vi "Custom Automation Tool.vi"(8 "error in (no error)":errorcluster) -> (0 "error out":errorcluster)   [LabVIEW 2023]
doc: "Presents an interface to either update a specification limit, or add a new one."
uses:
  CTLs/Step.ctl
  CTLs/Step Type.ctl
  <vilib>/Utility/config.llb/Config Data RefNum.ctl
  <vilib>/Utility/miscctls.llb/LVRowAndColumnUnsignedTypeDef.ctl
  CTLs/FGV Actions.ctl
  bd503c13-d10c-440e-ab5e-4e60baef5deb.vi
  cc7d3372-ed48-481f-8659-91fce09351ce.vi
  <vilib>/Utility/config.llb/Write Key (String).vi
  <vilib>/Utility/config.llb/Read Key (String).vi
  <userlib>/_MGI/Application Control/MGI Gray if/MGI Gray if False.vi
  <vilib>/Utility/inputDevices.llb/keyboardAcquire.vi
  <vilib>/Utility/inputDevices.llb/closeKeyboard.vi
  <vilib>/Utility/config.llb/NI_LVConfig.lvlib
  SubVIs/FaKI State Machine/FaKI State Machine.lvlib
panel:
  in  "Settings":bool
  in  "Export":bool
  in  "Import":bool
  out "Application Hotkey":string
  in  "Delete":bool
  in  "Start/Stop":bool
  in  "N":i32 caption="Times to Repeat\n(-1 = indefinitely)" min=-1
  in  "Activation Type":enum32{"Hotkey", "Automatic"}(radio)
  out "Menu":bool
  out "Row":i32
  in  "Add Step 2":bool
  in  "Dbl Click":T1
  out "Table":string[][](table)
  in  "Clear Profile":bool
  in  "Delete Step":bool
  in  "Insert Step":bool
  in  "Add Step":bool
  in  "Modify Step":bool
  in  "Close":bool
  in  "Save":bool
  in  "Restore":bool
  in  "Help":bool
  in  "Macro Name":string(combo)
  # "Table has double-click functionality"
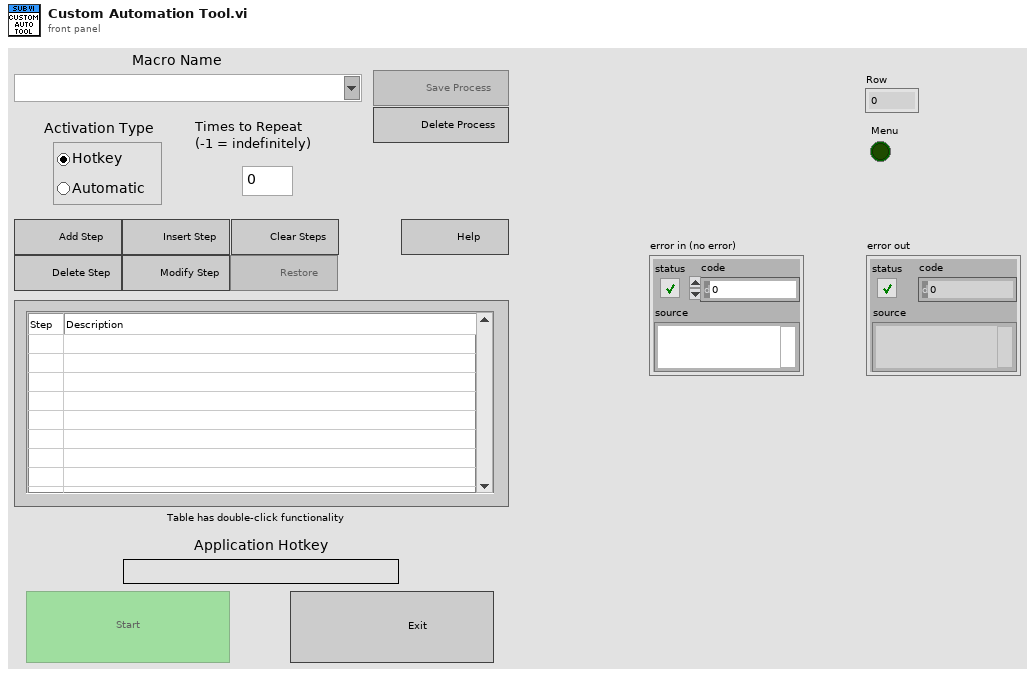
[diagram p1: front panel]
types:
  T1 = cluster{"Insert Before":bool, "Insert After":bool, "Modify":bool, "Delete":bool}
  T2 = typedef "LVPoint32TypeDef.ctl" = cluster{"Horizontal":i32, "Vertical":i32}
  T3 = typedef "LVRowAndColumnTypeDef.ctl" = cluster{"Row":i32, "Column":i32}
  T4 = enum32{"Invalid", "Standard", "Closed", "Hidden", "Minimized", "Maximized"}
  T5 = enum32{"invalid app kind", "Development System", "Run Time System", "Student Edition", "Embedded LabVIEW", "Evaluation", "Custom"}
  T6 = enum8{"Enabled", "Disabled", "Disabled and Grayed Out"}
  T7 = typedef "Step.ctl" = cluster{"Type":T8, "Coords":cluster{"x":i32, "y":i32}, "Delay":i32, "Key":u8, "Repeat":i32, "RClick?":bool}
  T8 = typedef "Step Type.ctl" = enum16{"Mouse Move", "Mouse Click", "Key Press", "Wait", "Mouse Down", "Mouse Up", "Key Down", "Key Up"}
  T9 = typedef "LVRowAndColumnUnsignedTypeDef.ctl" = cluster{"Row":u32, "Column":u32}
  T10 = cluster{"Steps":T7[], "Activation Type":enum32{"Hotkey", "Automatic"}, "N":i32}
  T11 = typedef "FGV Actions.ctl" = enum16{"Read", "Write"}
  T12 = typedef "NI_LVConfig.lvlib/Config Data RefNum.ctl" = refnum<k1>
  T13 = cluster{"Core":cluster{"Current VI Reference":refnum<vi>, "Close Panel on Exit?":bool}, "Steps":T7[], "Refs":refnum<vi>[], "Config":T12, "Step":i32, "n":i32, "Hotkey":enum16{"0", "1", "2", "3", "4", "5", "6", "7", "8", "9", "A", "B", "C", "D", "E", "F", "G", "H", "I", "J", "K", "L", "M", "N", "O", "P", "Q", "R", "S", "T", "U", "V", "W", "X", "Y", "Z", "F1", "F2", "F3", "F4", "F5", "F6", "F7", "F8", "F9", "F10", "F11", "F12", "F13", "F14", "F15", "ADD", "BACK", "BACKSLASH", "CAPITAL", "COMMA", "DECIMAL", "DELETE", "DIVIDE", "DOWN", "END", "EQUALS", "ESCAPE", "GRAVE (`)", "HOME", "INSERT", "LBRACKET", "LCONTROL", "LEFT", "L ALT", "LSHIFT", "LWIN", "MINUS", "MULTIPLY", "NEXT", "NUMLOCK", "NUMPAD_0", "NUMPAD_1", "NUMPAD_2", "NUMPAD_3", "NUMPAD_4", "NUMPAD_5", "NUMPAD_6", "NUMPAD_7", "NUMPAD_8", "NUMPAD_9", "PAUSE", "PERIOD", "PRIOR (PG UP)", "RBRACKET", "RCONTROL", "RETURN", "RIGHT", "R ALT", "RSHIFT", "RWIN", "SCROLL", "SEMICOLON", "SLASH", "SPACE", "SUBTRACT", "TAB", "UP", "ENTER (num pad)", "' (quote)"}[], "FP CTLs":cluster{"Name":string, "Type":enum32{"Hotkey", "Automatic"}, "N":i32}, "Keyboard":refnum<k1>}
  T14 = cluster{"Name":string, "Type":enum32{"Hotkey", "Automatic"}, "N":i32}
  T15 = enum16{"0", "1", "2", "3", "4", "5", "6", "7", "8", "9", "A", "B", "C", "D", "E", "F", "G", "H", "I", "J", "K", "L", "M", "N", "O", "P", "Q", "R", "S", "T", "U", "V", "W", "X", "Y", "Z", "F1", "F2", "F3", "F4", "F5", "F6", "F7", "F8", "F9", "F10", "F11", "F12", "F13", "F14", "F15", "ADD", "BACK", "BACKSLASH", "CAPITAL", "COMMA", "DECIMAL", "DELETE", "DIVIDE", "DOWN", "END", "EQUALS", "ESCAPE", "GRAVE (`)", "HOME", "INSERT", "LBRACKET", "LCONTROL", "LEFT", "L ALT", "LSHIFT", "LWIN", "MINUS", "MULTIPLY", "NEXT", "NUMLOCK", "NUMPAD_0", "NUMPAD_1", "NUMPAD_2", "NUMPAD_3", "NUMPAD_4", "NUMPAD_5", "NUMPAD_6", "NUMPAD_7", "NUMPAD_8", "NUMPAD_9", "PAUSE", "PERIOD", "PRIOR (PG UP)", "RBRACKET", "RCONTROL", "RETURN", "RIGHT", "R ALT", "RSHIFT", "RWIN", "SCROLL", "SEMICOLON", "SLASH", "SPACE", "SUBTRACT", "TAB", "UP", "ENTER (num pad)", "' (quote)"}[]
  T16 = cluster{"Current VI Reference":refnum<vi>, "Close Panel on Exit?":bool}
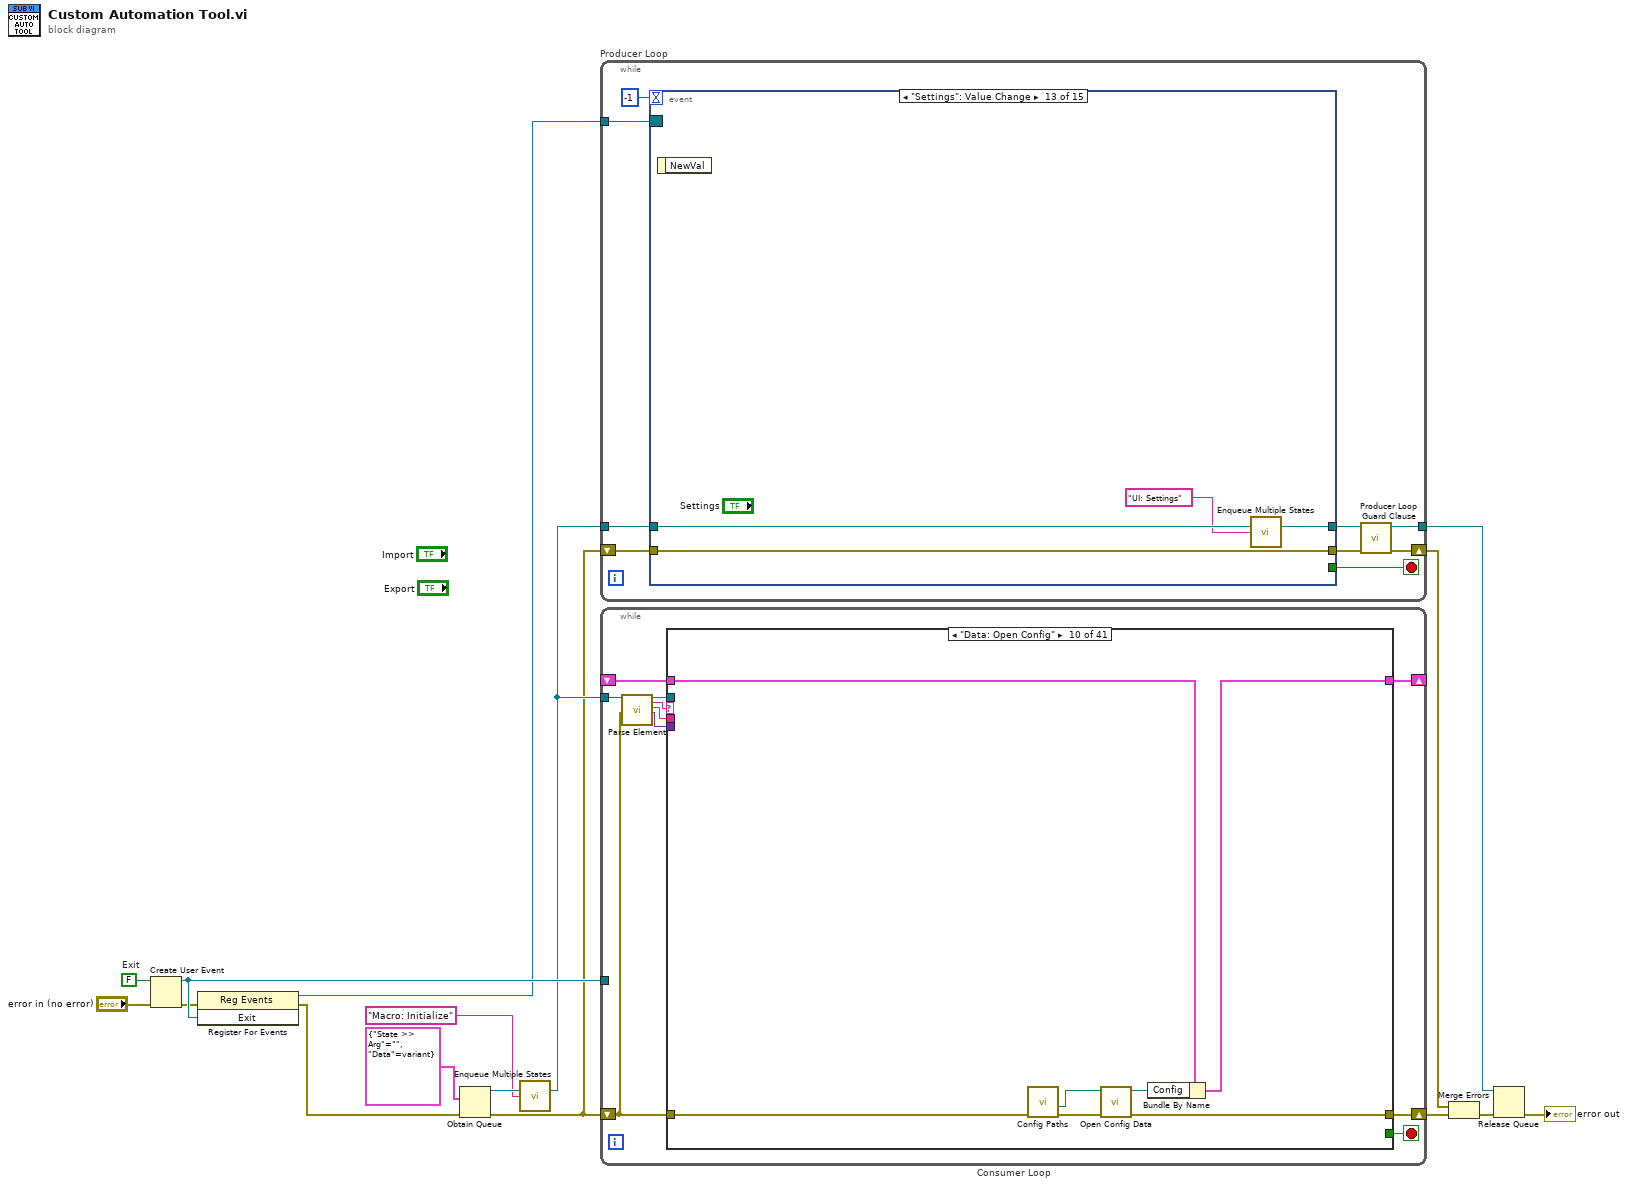
[diagram p0: block diagram]
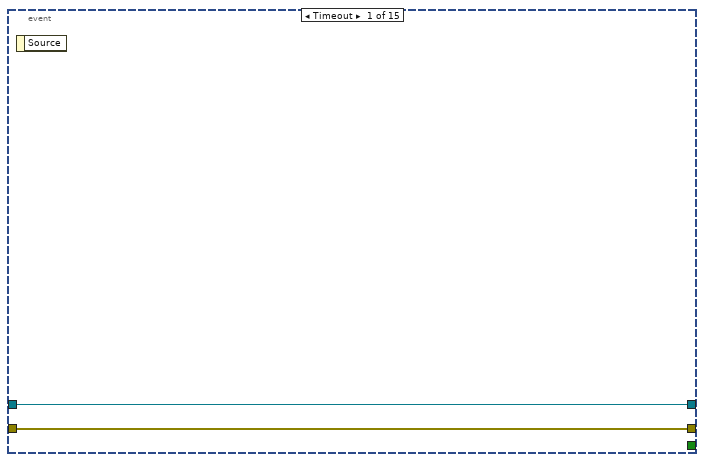
[diagram p2: hidden frame]
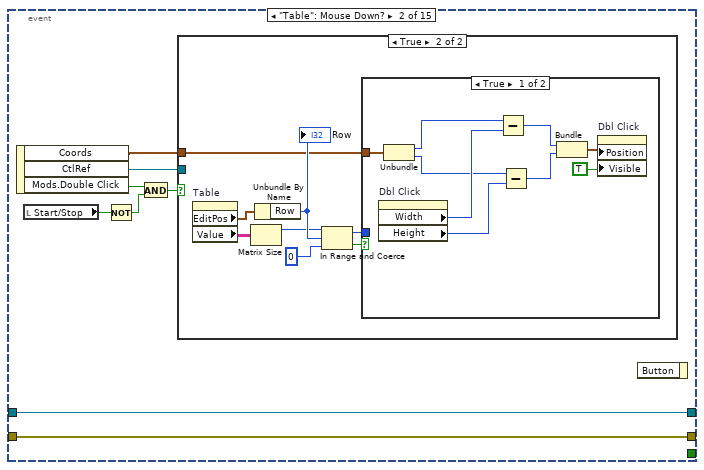
[diagram p3: hidden frame]
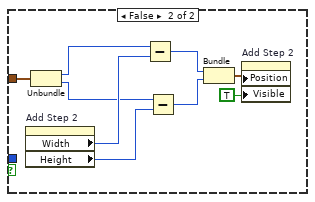
[diagram p5: hidden frame]
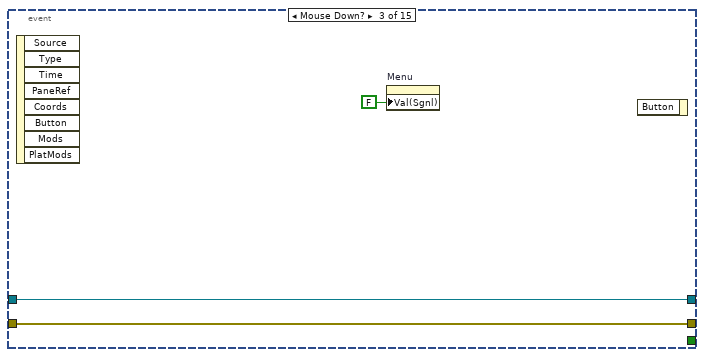
[diagram p6: hidden frame]
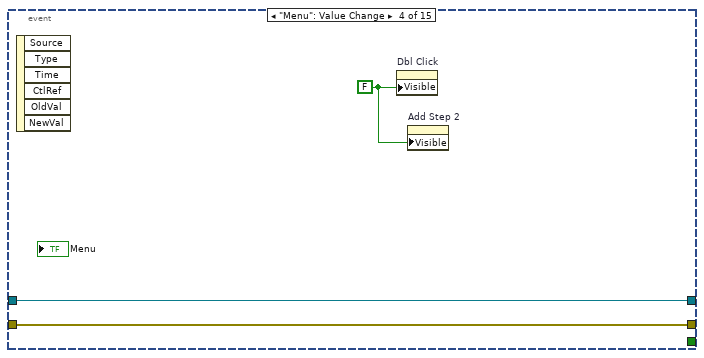
[diagram p7: hidden frame]
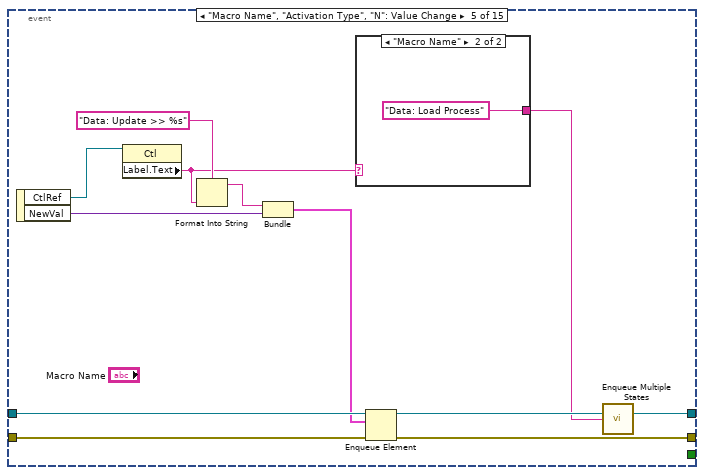
[diagram p8: hidden frame]
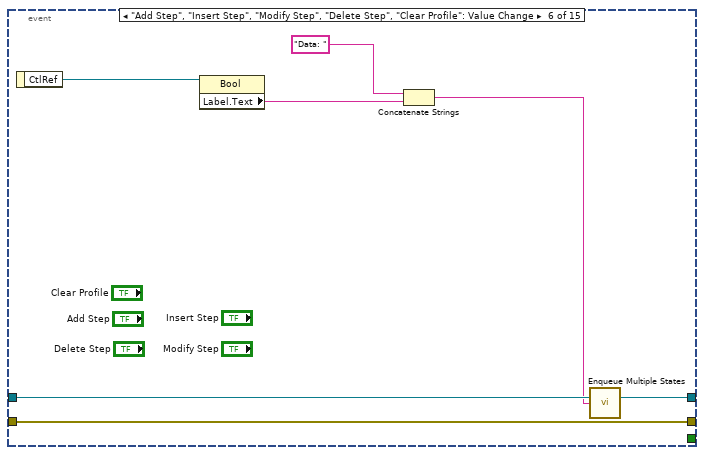
[diagram p10: hidden frame]
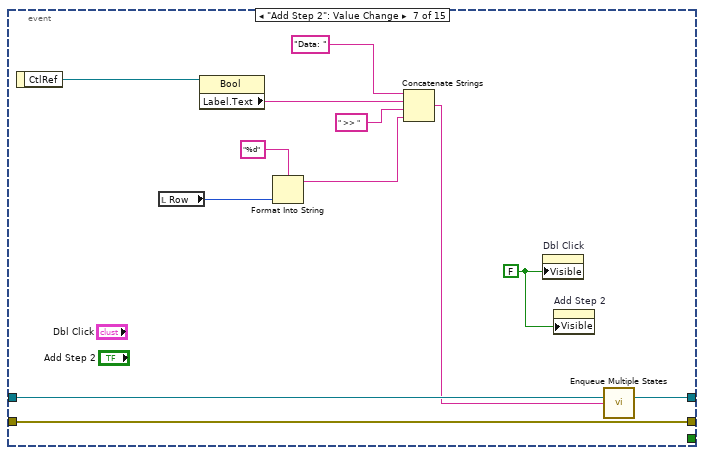
[diagram p11: hidden frame]
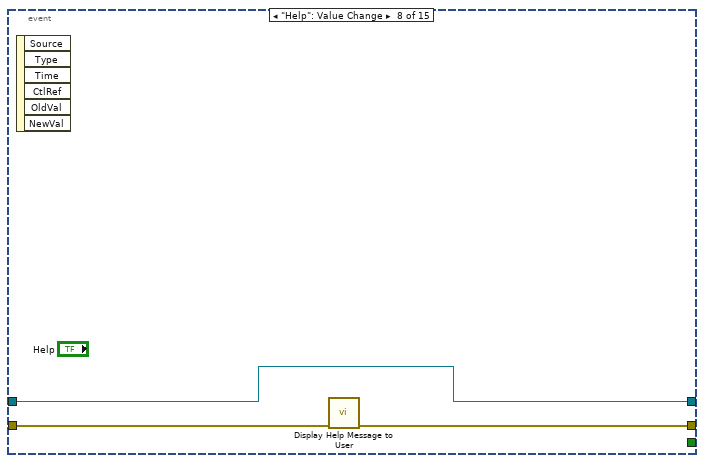
[diagram p12: hidden frame]
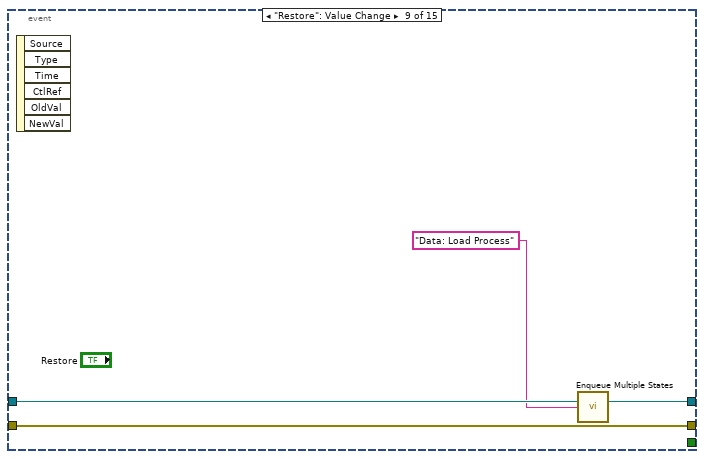
[diagram p13: hidden frame]
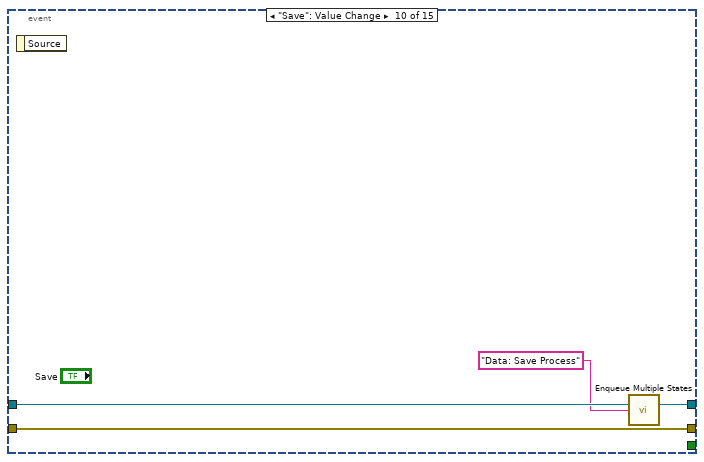
[diagram p14: hidden frame]
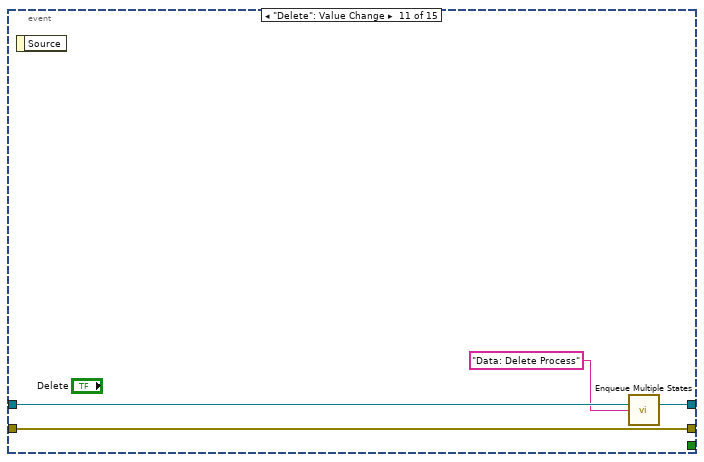
[diagram p15: hidden frame]
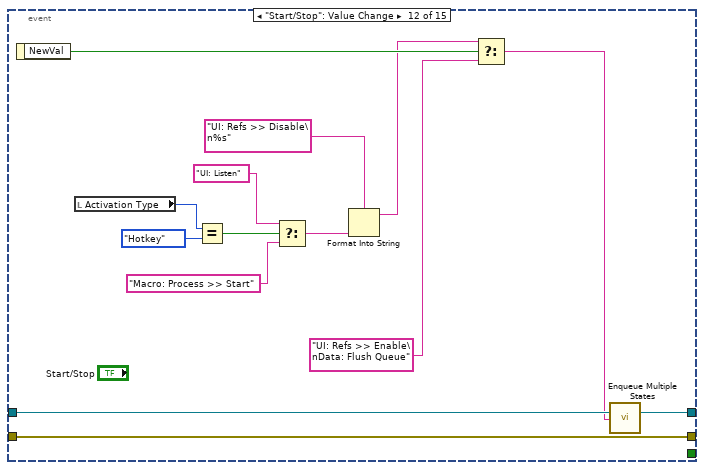
[diagram p16: hidden frame]
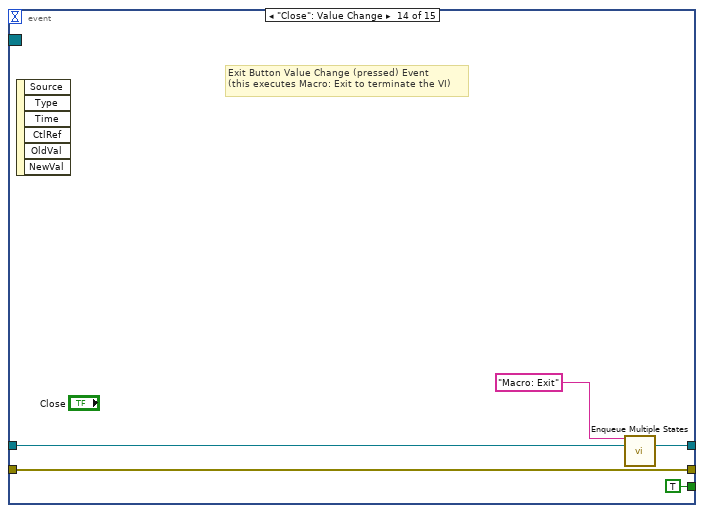
[diagram p17: hidden frame]
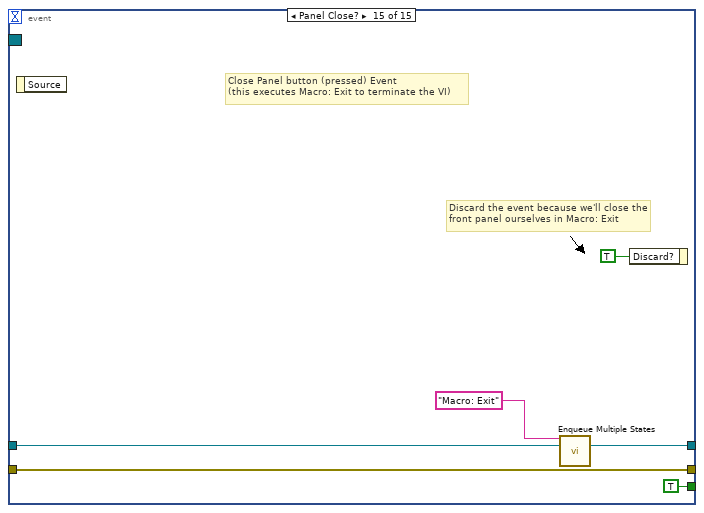
[diagram p18: hidden frame]
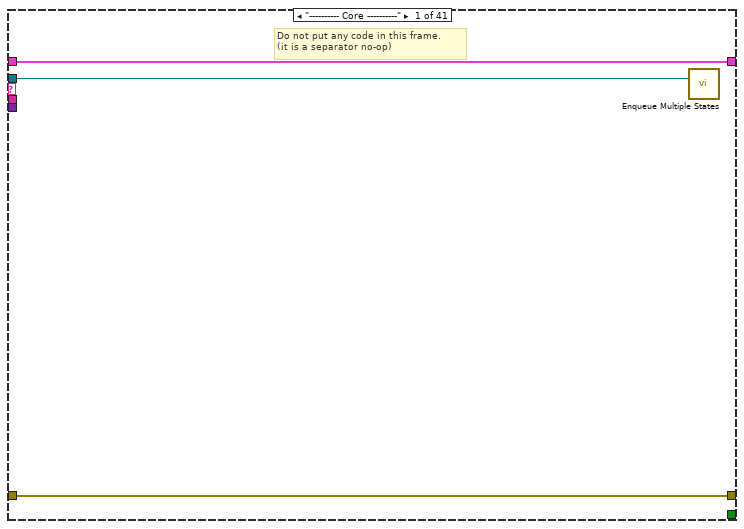
[diagram p19: hidden frame]
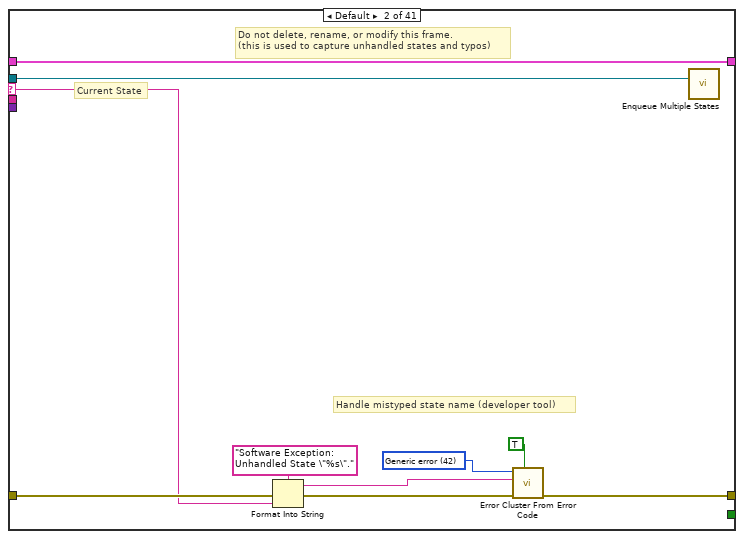
[diagram p20: hidden frame]
diagram:
  w13 = FALSE  # Exit
  n1 = Create User Event(user event datatype=w13, error in="error in (no error)") -> (user event=w16:refnum<user-event>, error out=w12:errorcluster)
  n2 = register-events(error in=w12, w16) -> (reference out=w15:refnum<event-registration>, error out=w14:errorcluster)  [unwired: 1 in]
  n3 = Obtain Queue(element data type=cluster{"State >> Arg":string, "Data":variant} {"State >> Arg"="", "Data"=variant}, error in (no error)=w14) -> (queue out=w6:refnum<queue>, error out=w3:errorcluster)  [unwired: 3 in, 1 out]
  n4 = call "Enqueue Multiple States.vi"("queue in"=w6, "State(s) at Back"="Macro: Initialize") -> ("queue out"=w7:refnum<queue>)  [unwired: 13 in]
  n5 = while "Producer Loop" {
    shift-right: [w25] -> w9
    shift-left: w3 -> [w23]
    tunnel: w15 -> [w19]
    tunnel: w7 -> [w21]
    tunnel: [w24] -> w11
    stop <- w18 stop-if-true
    n6 = event shown="[12] \"Settings\": Value Change" {
      selector: w19 -> [_ _ _ _ _ _ _ _ _ _ _ _ _ _ _]
      dyn-events: _ -> [_ _ _ _ _ _ _ _ _ _ _ _ _ _ _]
      timeout: -1 ("Timeout") -> [_ _ _ _ _ _ _ _ _ _ _ _ _ _ _]
      tunnel: [w27 w35 w64 w67 w75 w87 w99 w101 w106 w110 w114 w128 w132 w137 w143] -> w22
      tunnel: w23 -> [w27 w35 w64 w67 w78 w87 w99 w102 w106 w110 w114 w128 w132 w137 w143]
      tunnel: w21 -> [w26 w32 w62 w65 w72 w83 w90 w100 w104 w109 w113 w116 w130 w135 w140]
      tunnel: [w26 w32 w62 w65 w77 w82 w89 w100 w105 w108 w112 w117 w131 w134 w139] -> w20
      tunnel: [_ _ _ _ _ _ _ _ _ _ _ _ _ TRUE TRUE] -> w18
      event Timeout {
        n7 = event-data() -> ()  [unwired: 1 in, 1 out]
      }
      event "Table": Mouse Down? {
        n8 = event-data() -> ("Coords"=w33:T2, "CtlRef"=w34:refnum<vi>, "Mods.Double Click"=w29:bool)  [unwired: 1 in]
        n9 = local read "Start/Stop"() -> (w31:bool)
        n10 = Not(x=w31) -> (.not. x?=w30:bool)
        n11 = And(x=w29, y=w30) -> (x .and. y?=w28:bool)
        n12 = case shown="True" w28 {
          tunnel: w34 -> [_ _]
          tunnel: w33 -> [_ w36]
          frame False {
          }
          frame True {
            n13 = property on="Table" class="Tbl (strict)"() -> ("EditPos"=w42:T3, "Value"=w43:string[][])  [unwired: 2 in, 2 out]
            n14 = Matrix Size(0:w43) -> (1:w40:i32)  [unwired: 1 out]
            n15 = Unbundle By Name(w42) -> ("Row"=w41:i32)
            "Row" <- w41
            n16 = In Range and Coerce(upper limit=w40, x=w41, lower limit=0) -> (coerced(x)=w37:i32, In Range?=w38:bool)
            n17 = case shown="True" w38 {
              tunnel: w37 -> [_ _]
              tunnel: w36 -> [w51 w60]
              frame True {
                n18 = property on="Dbl Click" class="Clust"() -> ("Width"=w49:u32, "Height"=w48:u32)  [unwired: 2 in, 2 out]
                n19 = Unbundle(w51) -> ("Horizontal"=w50:i32, "Vertical"=w47:i32)
                n20 = Subtract(x=w50, y=w49) -> (x-y=w45:u32)
                n21 = Subtract(x=w47, y=w48) -> (x-y=w46:u32)
                n22 = Bundle(w45, w46) -> (w44:cluster{u32, u32})  [unwired: 1 in]
                n23 = property on="Dbl Click" class="Clust"("Position"=w44, "Visible"=TRUE) -> ()  [unwired: 2 in, 2 out]
              }
              frame False {
                n24 = property on="Add Step 2" class="Bool"() -> ("Width"=w58:u32, "Height"=w57:u32)  [unwired: 2 in, 2 out]
                n25 = Unbundle(w60) -> ("Horizontal"=w59:i32, "Vertical"=w56:i32)
                n26 = Subtract(x=w59, y=w58) -> (x-y=w54:u32)
                n27 = Subtract(x=w56, y=w57) -> (x-y=w55:u32)
                n28 = Bundle(w54, w55) -> (w53:cluster{u32, u32})  [unwired: 1 in]
                n29 = property on="Add Step 2" class="Bool"("Position"=w53, "Visible"=TRUE) -> ()  [unwired: 2 in, 2 out]
              }
            }
          }
        }
        n30 = event-data() -> ()  [unwired: 2 in, 1 out]
      }
      event Mouse Down? {
        n31 = event-data() -> ()  [unwired: 1 in, 8 out]
        n32 = property on="Menu" class="Bool (strict)"("Val(Sgnl)"=FALSE ("Value (Signaling)")) -> ()  [unwired: 2 in, 2 out]
        n33 = event-data() -> ()  [unwired: 2 in, 1 out]
      }
      event "Menu": Value Change {
        w66 = FALSE ("Visible")
        n34 = event-data() -> ()  [unwired: 1 in, 6 out]
        n35 = property on="Dbl Click" class="Clust"("Visible"=w66) -> ()  [unwired: 2 in, 2 out]
        n36 = property on="Add Step 2" class="Bool"("Visible"=w66) -> ()  [unwired: 2 in, 2 out]
      }
      event "Macro Name", "Activation Type", "N": Value Change {
        n37 = event-data() -> ("CtlRef"=w74:refnum<vi>, "NewVal"=w70:variant)  [unwired: 1 in]
        n38 = property class="Ctl"(reference=w74) -> ("Label.Text"=w69:string)  [unwired: 1 in, 2 out]
        n39 = Format Into String(format string="Data: Update >> %s", w69) -> (resulting string=w71:string)  [unwired: 2 in, 1 out]
        n40 = Bundle(w71, "NewVal"=w70) -> (w68:cluster{string, "NewVal":variant})  [unwired: 1 in]
        n41 = case shown="\"Macro Name\"" w69 {
          tunnel: [_ "Data: Load Process" ("string")] -> w76
          frame "False", Default {
          }
          frame "Macro Name" {
          }
        }
        n42 = Enqueue Element(queue=w72, element=w68, error in (no error)=w78) -> (queue out=w79:refnum<queue>, error out=w75:errorcluster)  [unwired: 1 in, 1 out]
        n43 = call "Enqueue Multiple States.vi"("queue in"=w79, "State(s) at Back"=w76) -> ("queue out"=w77:refnum<queue>)  [unwired: 13 in]
      }
      event "Add Step", "Insert Step", "Modify Step", "Delete Step", "Clear Profile": Value Change {
        n44 = event-data() -> ("CtlRef"=w86:refnum<vi>)  [unwired: 1 in]
        n45 = property class="Bool"(reference=w86) -> ("Label.Text"=w84:string)  [unwired: 1 in, 2 out]
        n46 = Concatenate Strings("Data: " ("State(s) at Back (\"\")"), w84) -> (w81:string)
        n47 = call "Enqueue Multiple States.vi"("queue in"=w83, "State(s) at Back"=w81) -> ("queue out"=w82:refnum<queue>)  [unwired: 13 in]
      }
      event "Dbl Click.Insert Before", "Dbl Click.Insert After", "Dbl Click.Modify", "Dbl Click.Delete", "Add Step 2": Value Change {
        w92 = FALSE ("Visible")
        n48 = event-data() -> ("CtlRef"=w98:refnum<vi>)  [unwired: 1 in]
        n49 = local read "Row"() -> (w91:i32)
        n50 = property class="Bool"(reference=w98) -> ("Label.Text"=w96:string)  [unwired: 1 in, 2 out]
        n51 = Format Into String(format string="%d", w91) -> (resulting string=w93:string)  [unwired: 2 in, 1 out]
        n52 = Concatenate Strings("Data: " ("State(s) at Back (\"\")"), w96, " >> " ("string"), w93) -> (w88:string)
        n53 = property on="Dbl Click" class="Clust"("Visible"=w92) -> ()  [unwired: 2 in, 2 out]
        n54 = property on="Add Step 2" class="Bool"("Visible"=w92) -> ()  [unwired: 2 in, 2 out]
        n55 = call "Enqueue Multiple States.vi"("queue in"=w90, "State(s) at Back"=w88) -> ("queue out"=w89:refnum<queue>)  [unwired: 13 in]
      }
      event "Help": Value Change {
        n56 = event-data() -> ()  [unwired: 1 in, 6 out]
        n57 = call "Display Help Message to User"("error in (no error)"=w102) -> ("error out"=w101:errorcluster)  [unwired: 9 in, 1 out]
      }
      event "Restore": Value Change {
        n58 = event-data() -> ()  [unwired: 1 in, 6 out]
        n59 = call "Enqueue Multiple States.vi"("queue in"=w104, "State(s) at Back"="Data: Load Process" ("State(s) at Back (\"\")")) -> ("queue out"=w105:refnum<queue>)  [unwired: 13 in]
      }
      event "Save": Value Change {
        n60 = event-data() -> ()  [unwired: 1 in, 1 out]
        n61 = call "Enqueue Multiple States.vi"("queue in"=w109, "State(s) at Back"="Data: Save Process" ("State(s) at Back (\"\")")) -> ("queue out"=w108:refnum<queue>)  [unwired: 13 in]
      }
      event "Delete": Value Change {
        n62 = event-data() -> ()  [unwired: 1 in, 1 out]
        n63 = call "Enqueue Multiple States.vi"("queue in"=w113, "State(s) at Back"="Data: Delete Process" ("State(s) at Back (\"\")")) -> ("queue out"=w112:refnum<queue>)  [unwired: 13 in]
      }
      event "Start/Stop": Value Change {
        n64 = event-data() -> ("NewVal"=w120:bool)  [unwired: 1 in]
        n65 = local read "Activation Type"() -> (w127:enum32{"Hotkey", "Automatic"})
        n66 = Equal?(x=w127, y=enum32{"Hotkey", "Automatic"}."Hotkey") -> (x = y?=w125:bool)
        n67 = Select(t="UI: Listen", s=w125, f="Macro: Process >> Start") -> (s? t:f=w122:string)
        n68 = Format Into String(format string="UI: Refs >> Disable\n%s" ("State(s) at Back (\"\")"), w122) -> (resulting string=w119:string)  [unwired: 2 in, 1 out]
        n69 = Select(t=w119, s=w120, f="UI: Refs >> Enable\nData: Flush Queue") -> (s? t:f=w115:string)
        n70 = call "Enqueue Multiple States.vi"("queue in"=w116, "State(s) at Back"=w115) -> ("queue out"=w117:refnum<queue>)  [unwired: 13 in]
      }
      event "Settings": Value Change {
        n71 = event-data() -> ()  [unwired: 1 in, 1 out]
        n72 = call "Enqueue Multiple States.vi"("queue in"=w130, "State(s) at Back"="UI: Settings" ("f")) -> ("queue out"=w131:refnum<queue>)  [unwired: 13 in]
      }
      event "Close": Value Change {
        # "Exit Button Value Change (pressed) Event\n(this executes Macro: Exit to terminate the VI)"
        n73 = event-data() -> ()  [unwired: 1 in, 6 out]
        n74 = call "Enqueue Multiple States.vi"("State(s) at Front"="Macro: Exit", "queue in"=w135) -> ("queue out"=w134:refnum<queue>)  [unwired: 13 in]
      }
      event Panel Close? {
        # "Discard the event because we'll close the front panel ourselves in Macro: Exit"
        # "Close Panel button (pressed) Event\n(this executes Macro: Exit to terminate the VI)"
        n75 = event-data() -> ()  [unwired: 1 in, 1 out]
        n76 = call "Enqueue Multiple States.vi"("State(s) at Front"="Macro: Exit", "queue in"=w140) -> ("queue out"=w139:refnum<queue>)  [unwired: 13 in]
        n77 = event-data("Discard?"=TRUE) -> ()  [unwired: 1 in, 1 out]
      }
    }
    n78 = call "Producer Loop Guard Clause.vi"("error in (no error)"=w22, "queue in"=w20) -> ("error out"=w25:errorcluster, "queue out"=w24:refnum<queue>)  [unwired: 8 in]
  }
  n79 = while "Consumer Loop" {
    shift-right: [w148] -> _
    shift-left: _ -> [w149]
    shift-right: [w151] -> w8
    shift-left: w3 -> [w152]
    tunnel: w7 -> [w153]
    tunnel: w16 -> [_]
    stop <- w150 stop-if-true
    n80 = call "Parse Element.vi"("queue in"=w153, "error in (no error)"=w152) -> ("queue out"=w147:refnum<queue>, "State"=w146:string, "Arg"=w145:string, "Data"=w144:variant)  [unwired: 14 in]
    n81 = case shown="\"Data: Open Config\"" w146 {
      selector: w146 -> [_ w158 _ _ _ _ _ _ _ _ _ _ _ _ _ _ _ _ _ _ _ _ _ _ _ _ _ _ _ _ _ _ _ _ _ _ _ _ _ _ _]
      tunnel: w147 -> [w154 w157 w167 w179 w186 w190 _ _ _ _ w258 w266 w274 w282 w290 w298 w309 w321 w332 w343 _ w395 _ w434 w440 w445 w454 w456 w465 _ w541 _ w566 w576 _ w592 w595 w600 w644 w651 w655]
      tunnel: w145 -> [_ _ _ w181 _ _ _ _ w225 _ _ _ _ _ _ w300 w312 w323 w334 _ _ _ _ _ _ _ _ w457 w466 _ _ w559 _ _ _ _ _ w603 _ _ _]
      tunnel: w149 -> [w155 w160 w173 w184 w189 w191 _ w209 w226 w253 w261 w267 w275 w283 w291 w301 w313 w324 w335 w345 w355 w392 w421 w435 w444 w446 w450 w460 w468 w540 w554 w558 w574 w579 w591 w593 w597 w599 w649 w652 w671]
      tunnel: [w156 w162 w177 errorcluster {"status"=FALSE, "code"=0, "source"=""} ("error out") w188 w192 w198 w211 w221 w254 w262 w270 w278 w286 w294 w304 w316 w327 w338 w348 w362 w401 w422 w436 w442 w447 w452 w458 w469 w538 w551 w557 w573 w580 w589 w594 w598 w604 w650 w653 w662] -> w151
      tunnel: w152 -> [w156 w161 w177 w183 w188 w192 w199 w211 w224 w255 w262 w270 w278 w286 w294 w304 w316 w327 w338 w348 w364 w406 w423 w436 w441 w447 w453 w459 w470 w539 w552 w557 w570 w581 w590 w594 w598 w604 w650 w653 w663]
      tunnel: [_ _ _ _ TRUE _ _ _ _ _ _ _ _ _ _ _ _ _ _ _ _ _ _ _ _ _ _ _ _ _ _ _ _ _ _ _ _ _ _ _ _] -> w150
      tunnel: [w155 w160 w178 w184 w189 w191 w206 w207 w222 w252 w260 w269 w277 w285 w293 w303 w315 w326 w337 w344 w361 w393 w421 w435 w444 w446 w449 w460 w468 w540 w554 w558 w574 w579 w591 w593 w597 w602 w649 w652 w671] -> w148
      tunnel: w144 -> [_ _ _ w180 _ _ _ _ w223 _ _ _ _ _ _ _ _ _ _ _ _ _ _ _ _ _ _ _ _ _ _ _ _ _ _ _ _ _ _ _ _]
      frame "---------- Core ----------" {
        # "Do not put any code in this frame.\n(it is a separator no-op)"
        n82 = call "Enqueue Multiple States.vi"("queue in"=w154) -> ()  [unwired: 14 in, 1 out]
      }
      frame Default {
        w165 = 42 items=["No error", "Argument error", "Memory is full", "Out of zone", "End of file", "File already open", "Generic file I/O error", "File not found", "File permission error", "Disk is full", "Duplicate path", "Too many files open", "System feature not enabled", "Resource file not found", "Cannot add resource", "Resource not found", "Image not found", "Image memory error", "Pen does not exist", "Config type invalid", "Config token not found", "Config parse error", "Config memory error", "Bad external code format", "Bad external code offset", "External code not present", "Null window", "Destroy window error", "Null menu", "Print aborted", "Bad print record", "Print driver error", "Windows error during printing", "Memory error during printing", "Print dialog error", "Generic print error", "Invalid device refnum", "Device not found", "Device parameter error", "Device unit error", "Cannot open device", "Device call aborted", "Generic error", "Cancelled by user", "Object ID too low", "Object ID too high", "Object not in heap", "Unknown heap", "Unknown object (invalid DefProc)", "Unknown object (DefProc not in table)", "Message out of range", "Invalid (null) method", "Unknown message", "Manager call not supported", "Bad address", "Network operation in progress", "Network operation timed out", "Connection is busy", "Network attribute not supported", "Network error", "Address in use", "System out of memory", "Connection aborted", "Connection refused", "Not connected", "Already connected", "Connection closed", "Initialization error (interapplication manager)", "Bad occurrence", "Wait on unbound occurrence handler", "Occurrence queue overflow", "Datalog type conflict", "Unused", "Unrecognized type (interapplication manager)", "Memory corrupt", "Failed to make temporary DLL", "Old CIN version", "Drag socket not found", "Failed to load drop-object", "Failed to register OLE object", "Failed to release OLE object", "Format specifier type mismatch", "Unknown format specifier", "Too few format specifiers", "Too many format specifiers", "Scan failed", "Newer CIN version", "Error converting to variant", "Runtime menu error", "Password tampered", "Variant attribute not found", "Incompatible variant data type", "Event data is not available", "Event Store is not present", "Occurrence is not found", "Event Queue is not created", "Event info is not available", "Refnum passed is NULL", "Error retrieving Class GUID", "Error retrieving CoClass GUID", "Error retrieving TypeLib GUID.", "Bad built application magic bytes.", "Specific driver is different from the specific driver associated with the Logical Name.", "There is no session opened to the class driver.", "Max Error", "MAX - Error with config objects", "MAX - Error loading configuration", "MAX - Group not supported"]
        # "Current State"
        # "Do not delete, rename, or modify this frame.\n(this is used to capture unhandled states and typos)"
        # "Handle mistyped state name (developer tool)"
        n83 = Format Into String(format string="Software Exception: Unhandled State \"%s\"." ("message"), error in=w161, w158) -> (resulting string=w164:string, error out=w163:errorcluster)  [unwired: 1 in]
        n84 = call <vilib>:"Error Cluster From Error Code.vi"("show call chain? (False)"=TRUE, "error in (no error)"=w163, "error message (\"\")"=w164, "error code (0)"=w165) -> ("error out"=w162:errorcluster)  [unwired: 5 in]
        n85 = call "Enqueue Multiple States.vi"("queue in"=w157) -> ()  [unwired: 14 in, 1 out]
      }
      frame "Initialize Core Data" {
        # "Do not delete, rename, or modify this frame.\n(this is used to determine panel behavior on exit)"
        # "originally closed?"
        # "exe?"
        # "If panel starts closed or is an EXE, then close it when we exit"
        n86 = property class="VI"() -> ("FP.State"=w170:T4)  [unwired: 2 in, 2 out]
        n87 = property class="App"() -> ("App.Kind"=w176:T5)  [unwired: 2 in, 2 out]
        n88 = control-ref of="Current VI Reference"() -> (w171:refnum<vi>)
        n89 = Equal?(x=w170, y=T4."Closed" ("Front Panel Window:State")) -> (x = y?=w168:bool)
        n90 = Equal?(x=w176, y=T5."Run Time System" ("Application:Kind")) -> (x = y?=w174:bool)
        n91 = Or(x=w168, y=w174) -> (x .or. y?=w172:bool)
        n92 = Bundle By Name(cluster=w173, "Core.Current VI Reference"=w171, "Core.Close Panel on Exit?"=w172) -> (w178:T13)
        n93 = call "Enqueue Multiple States.vi"("queue in"=w167) -> ()  [unwired: 14 in, 1 out]
      }
      frame "Error Handler" {
        # "Unhandled Error -- Display it"
        # "Handle any errors here.\nYou can also output any states to clean-up after errors occur"
        # "Clear error"
        n94 = call "Build Error Message.vi"("error in (no error)"=w183, "Data"=w180, "Arg"=w181) -> ("error out"=w182:errorcluster)  [unwired: 8 in]
        n95 = call <vilib>:"General Error Handler.vi"("error in (no error)"=w182) -> ()  [unwired: 10 in, 5 out]
        n96 = call "Enqueue Multiple States.vi"("queue in"=w179) -> ()  [unwired: 14 in, 1 out]
      }
      frame "Exit" {
        # "Do not put any code in this frame.\n(No errors that occur here will be handled.)"
        n97 = call "Enqueue Multiple States.vi"("queue in"=w186) -> ()  [unwired: 14 in, 1 out]
      }
      frame "---------- Data ----------" {
        # "Do not put any code in this frame.\n(It is a separator no-op. You can make a copy of this frame to create a new Data frame)"
        n98 = call "Enqueue Multiple States.vi"("queue in"=w190) -> ()  [unwired: 14 in, 1 out]
      }
      frame "Data: Initialize" {
        w193 = T14 {"Name"="", "Type"=enum."Hotkey", "N"=0}  # FP CTLs
        w195 = T15 [] items=["0", "1", "2", "3", "4", "5", "6", "7", "8", "9", "A", "B", "C", "D", "E", "F", "G", "H", "I", "J", "K", "L", "M", "N", "O", "P", "Q", "R", "S", "T", "U", "V", "W", "X", "Y", "Z", "F1", "F2", "F3", "F4", "F5", "F6", "F7", "F8", "F9", "F10", "F11", "F12", "F13", "F14", "F15", "ADD", "BACK", "BACKSLASH", "CAPITAL", "COMMA", "DECIMAL", "DELETE", "DIVIDE", "DOWN", "END", "EQUALS", "ESCAPE", "GRAVE (`)", "HOME", "INSERT", "LBRACKET", "LCONTROL", "LEFT", "L ALT", "LSHIFT", "LWIN", "MINUS", "MULTIPLY", "NEXT", "NUMLOCK", "NUMPAD_0", "NUMPAD_1", "NUMPAD_2", "NUMPAD_3", "NUMPAD_4", "NUMPAD_5", "NUMPAD_6", "NUMPAD_7", "NUMPAD_8", "NUMPAD_9", "PAUSE", "PERIOD", "PRIOR (PG UP)", "RBRACKET", "RCONTROL", "RETURN", "RIGHT", "R ALT", "RSHIFT", "RWIN", "SCROLL", "SEMICOLON", "SLASH", "SPACE", "SUBTRACT", "TAB", "UP", "ENTER (num pad)", "' (quote)"]  # Hotkey
        w197 = refnum<k1> refnum items=["KEYBOARD"]  # Keyboard
        w201 = 0  # n
        w202 = 0  # Step
        w203 = T12 refnum items=["config data"]  # Config
        w204 = T7[] []  # Steps
        w194 = refnum<vi>[] []  # Refs
        w205 = T16 {"Current VI Reference"=refnum, "Close Panel on Exit?"=FALSE}  # Core
        # "Initialize the shift-register data, here.\n(data names are defined by what you wire into the bundle function)"
        n99 = call <vilib>:"Intialize Keyboard.vi"("error in (no error)"=w199) -> ("error out"=w198:errorcluster, "device ID"=w200:refnum<k1>)  [unwired: 9 in]
        n100 = Type Cast(type=w197, x=w200) -> (*(type *) &x=w196:refnum<k1>)
        n101 = Bundle("Core"=w205, "Steps"=w204, "Refs"=w194, "Config"=w203, "Step"=w202, "n"=w201, "Hotkey"=w195, "FP CTLs"=w193, "Keyboard"=w196) -> (w206:T13)  [unwired: 1 in]
      }
      frame "Data: Bundle Refs" {
        n102 = control-ref of="Activation Type"() -> (w214:refnum<vi>)
        n103 = control-ref of="Macro Name"() -> (w212:refnum<vi>)
        n104 = control-ref of="Add Step"() -> (w220:refnum<vi>)
        n105 = control-ref of="Delete Step"() -> (w218:refnum<vi>)
        n106 = control-ref of="Insert Step"() -> (w217:refnum<vi>)
        n107 = control-ref of="Modify Step"() -> (w219:refnum<vi>)
        n108 = control-ref of="Save"() -> (w216:refnum<vi>)
        n109 = control-ref of="Clear Profile"() -> (w215:refnum<vi>)
        n110 = control-ref of="Delete"() -> (w210:refnum<vi>)
        n111 = control-ref of="N"() -> (w213:refnum<vi>)
        n112 = Build Array(w220, w218, w217, w219, w216, w215, w214, w213, w212, w210) -> (w208:refnum<vi>[])
        n113 = Bundle By Name(cluster=w209, "Refs"=w208) -> (w207:T13)
      }
      frame "Data: Update" {
        n114 = case shown="\"Macro Name\"" w225 {
          tunnel: w226 -> [w227 w232 w240 w247]
          tunnel: w224 -> [w228 w236 w243 w250]
          tunnel: w223 -> [_ w235 w242 w249]
          tunnel: [w227 w231 w239 w246] -> w222
          tunnel: [w228 w230 w238 w245] -> w221
          frame "False", Default {
          }
          frame "Macro Name" {
            n115 = Variant To Data(error in=w236, type="", Variant=w235) -> (data=w233:string, error out=w230:errorcluster)
            n116 = property on="Restore" class="Bool"("DisabledEnum"=T6."Disabled and Grayed Out" ("Disabled")) -> ()  [unwired: 2 in, 2 out]
            n117 = Bundle By Name(cluster=w232, "FP CTLs.Name"=w233) -> (w231:T13)
          }
          frame "Activation Type" {
            n118 = Variant To Data(error in=w243, type=enum32{"Hotkey", "Automatic"}."Hotkey" ("FP CTLs.Type"), Variant=w242) -> (data=w241:enum32{"Hotkey", "Automatic"}, error out=w238:errorcluster)
            n119 = Bundle By Name(cluster=w240, "FP CTLs.Type"=w241) -> (w239:T13)
          }
          frame "N" {
            n120 = Variant To Data(error in=w250, type=0 ("FP CTLs.N"), Variant=w249) -> (data=w248:i32, error out=w245:errorcluster)
            n121 = Bundle By Name(cluster=w247, "FP CTLs.N"=w248) -> (w246:T13)
          }
        }
      }
      frame "Data: Open Config" {
        n122 = call "Config Paths.vi"("error in (no error)"=w255) -> ("error out"=w257:errorcluster, "Process Config"=w251:path)  [unwired: 7 in, 2 out]
        n123 = call <vilib>:"Open Config Data.vi"("error in (no error)"=w257, "configuration file path"=w251) -> ("error out"=w254:errorcluster, "refnum"=w256:T12)  [unwired: 7 in, 1 out]
        n124 = Bundle By Name(cluster=w253, "Config"=w256) -> (w252:T13)
      }
      frame "Data: Add Step" {
        n125 = in-place {
          n126 = in-place-cluster #1(w261) -> ("Steps"=w265:T7[])
          n127 = call "Alter Macro.vi"("Action"=enum16{"Add", "Insert", "Modify", "Delete"}."Add", "Steps in"=w265) -> ("Steps out"=w264:T7[])  [unwired: 9 in]
          n128 = in-place-cluster #1("Steps"=w264) -> (w260:T13)
        }
        n129 = call "Enqueue Multiple States.vi"("queue in"=w258, "State(s) at Back"="UI: Display Process" ("State(s) at Back (\"\")")) -> ()  [unwired: 13 in, 1 out]
      }
      frame "Data: Insert Step" {
        n130 = in-place {
          n131 = in-place-cluster #2(w267) -> ("Steps"=w273:T7[])
          n132 = call "Alter Macro.vi"("Action"=enum16{"Add", "Insert", "Modify", "Delete"}."Insert", "Steps in"=w273) -> ("Steps out"=w272:T7[])  [unwired: 9 in]
          n133 = in-place-cluster #2("Steps"=w272) -> (w269:T13)
        }
        n134 = call "Enqueue Multiple States.vi"("queue in"=w266, "State(s) at Back"="UI: Display Process" ("State(s) at Back (\"\")")) -> ()  [unwired: 13 in, 1 out]
      }
      frame "Data: Modify Step" {
        n135 = in-place {
          n136 = in-place-cluster #3(w275) -> ("Steps"=w281:T7[])
          n137 = call "Alter Macro.vi"("Action"=enum16{"Add", "Insert", "Modify", "Delete"}."Modify", "Steps in"=w281) -> ("Steps out"=w280:T7[])  [unwired: 9 in]
          n138 = in-place-cluster #3("Steps"=w280) -> (w277:T13)
        }
        n139 = call "Enqueue Multiple States.vi"("queue in"=w274, "State(s) at Back"="UI: Display Process" ("State(s) at Back (\"\")")) -> ()  [unwired: 13 in, 1 out]
      }
      frame "Data: Delete Step" {
        n140 = in-place {
          n141 = in-place-cluster #4(w283) -> ("Steps"=w289:T7[])
          n142 = call "Alter Macro.vi"("Action"=enum16{"Add", "Insert", "Modify", "Delete"}."Delete", "Steps in"=w289) -> ("Steps out"=w288:T7[])  [unwired: 9 in]
          n143 = in-place-cluster #4("Steps"=w288) -> (w285:T13)
        }
        n144 = call "Enqueue Multiple States.vi"("queue in"=w282, "State(s) at Back"="UI: Display Process" ("State(s) at Back (\"\")")) -> ()  [unwired: 13 in, 1 out]
      }
      frame "Data: Add Step 2" {
        n145 = in-place {
          n146 = in-place-cluster #5(w291) -> ("Steps"=w297:T7[])
          n147 = call "Alter Macro V2.vi"("Action"=enum16{"Add", "Insert", "Modify", "Delete"}."Add", "Steps in"=w297) -> ("Steps out"=w296:T7[])  [unwired: 9 in]
          n148 = in-place-cluster #5("Steps"=w296) -> (w293:T13)
        }
        n149 = call "Enqueue Multiple States.vi"("queue in"=w290, "State(s) at Back"="UI: Display Process" ("State(s) at Back (\"\")")) -> ()  [unwired: 13 in, 1 out]
      }
      frame "Data: Insert Before" {
        n150 = Decimal String To Number(string=w300) -> (number=w299:i32)  [unwired: 2 in, 1 out]
        n151 = in-place {
          in-place-border: w299 -> [w305]
          n152 = in-place-cluster #6(w301) -> ("Steps"=w308:T7[])
          n153 = call "Alter Macro V2.vi"("Action"=enum16{"Add", "Insert", "Modify", "Delete"}."Insert", "Step"=w305, "Steps in"=w308) -> ("Steps out"=w307:T7[])  [unwired: 8 in]
          n154 = in-place-cluster #6("Steps"=w307) -> (w303:T13)
        }
        n155 = call "Enqueue Multiple States.vi"("queue in"=w298, "State(s) at Back"="UI: Display Process" ("State(s) at Back (\"\")")) -> ()  [unwired: 13 in, 1 out]
      }
      frame "Data: Insert After" {
        n156 = Decimal String To Number(string=w312) -> (number=w311:i32)  [unwired: 2 in, 1 out]
        n157 = Increment(x=w311) -> (x+1=w310:i32)
        n158 = in-place {
          in-place-border: w310 -> [w317]
          n159 = in-place-cluster #7(w313) -> ("Steps"=w320:T7[])
          n160 = call "Alter Macro V2.vi"("Action"=enum16{"Add", "Insert", "Modify", "Delete"}."Insert", "Step"=w317, "Steps in"=w320) -> ("Steps out"=w319:T7[])  [unwired: 8 in]
          n161 = in-place-cluster #7("Steps"=w319) -> (w315:T13)
        }
        n162 = call "Enqueue Multiple States.vi"("queue in"=w309, "State(s) at Back"="UI: Display Process" ("State(s) at Back (\"\")")) -> ()  [unwired: 13 in, 1 out]
      }
      frame "Data: Modify" {
        n163 = Decimal String To Number(string=w323) -> (number=w322:i32)  [unwired: 2 in, 1 out]
        n164 = in-place {
          in-place-border: w322 -> [w328]
          n165 = in-place-cluster #8(w324) -> ("Steps"=w331:T7[])
          n166 = call "Alter Macro V2.vi"("Action"=enum16{"Add", "Insert", "Modify", "Delete"}."Modify", "Step"=w328, "Steps in"=w331) -> ("Steps out"=w330:T7[])  [unwired: 8 in]
          n167 = in-place-cluster #8("Steps"=w330) -> (w326:T13)
        }
        n168 = call "Enqueue Multiple States.vi"("queue in"=w321, "State(s) at Back"="UI: Display Process" ("State(s) at Back (\"\")")) -> ()  [unwired: 13 in, 1 out]
      }
      frame "Data: Delete" {
        n169 = Decimal String To Number(string=w334) -> (number=w333:i32)  [unwired: 2 in, 1 out]
        n170 = in-place {
          in-place-border: w333 -> [w339]
          n171 = in-place-cluster #9(w335) -> ("Steps"=w342:T7[])
          n172 = call "Alter Macro V2.vi"("Action"=enum16{"Add", "Insert", "Modify", "Delete"}."Delete", "Step"=w339, "Steps in"=w342) -> ("Steps out"=w341:T7[])  [unwired: 8 in]
          n173 = in-place-cluster #9("Steps"=w341) -> (w337:T13)
        }
        n174 = call "Enqueue Multiple States.vi"("queue in"=w332, "State(s) at Back"="UI: Display Process" ("State(s) at Back (\"\")")) -> ()  [unwired: 13 in, 1 out]
      }
      frame "Data: Clear Profile" {
        n175 = call "Display Message to User"() -> ("OK"=w346:bool)  [unwired: 10 in, 1 out]
        n176 = case shown="True" w346 {
          tunnel: w345 -> [w349 w353]
          tunnel: [w349 w352] -> w344
          frame False {
          }
          frame True {
            n177 = Bundle By Name(cluster=w353, "Steps"=T7[] []) -> (w352:T13)
            n178 = property on="Table" class="Tbl (strict)"("Index Values"=T9 {"Row"=0, "Column"=0}) -> ()  [unwired: 2 in, 2 out]
          }
        }
        n179 = call "Enqueue Multiple States.vi"("queue in"=w343, "State(s) at Back"="UI: Display Process" ("State(s) at Back (\"\")")) -> ()  [unwired: 13 in, 1 out]
      }
      frame "Data: Save Process" {
        n180 = local read "Macro Name"() -> (w360:string)
        n181 = Unbundle By Name(w355) -> ("Config"=w356:T12)
        n182 = call <vilib>:"Get Section Names.vi"("refnum"=w356) -> ("error out"=w359:errorcluster, "section names"=w357:string[])  [unwired: 8 in, 1 out]
        n183 = Unbundle By Name(w355) -> ("Steps"=w368:T7[])
        n184 = Search 1D Array(1D array=w357, element=w360) -> (index of element=w358:i32)  [unwired: 1 in]
        n185 = Bundle("Steps"=w368, "Activation Type"="Activation Type", "N"="N") -> (w365:T10)  [unwired: 1 in]
        n186 = case shown="0, Default" w358 {
          tunnel: w359 -> [w389 w390]
          tunnel: [w388 w390] -> _
          tunnel: [w387 TRUE ("Overwrite")] -> w354
          frame 0, Default {
            n187 = call "Overwrite?"("error in (no error)"=w389) -> ("error out"=w388:errorcluster, "Overwrite"=w387:bool)  [unwired: 9 in]
          }
          frame -1 {
          }
        }
        n188 = Flatten To String(anything=w365) -> (data string=w363:string)  [unwired: 3 in, 2 out]
        n189 = case shown="True" w354 {
          tunnel: w364 -> [w369 w375]
          tunnel: w363 -> [_ w374]
          tunnel: [w369 w373] -> w362
          tunnel: [w370 w372] -> w361
          tunnel: w355 -> [w370 w371]
          frame False {
          }
          frame True {
            n190 = in-place {
              in-place-border: w375 -> [w384]
              in-place-border: w374 -> [w383]
              in-place-border: [w377] -> w373
              n191 = in-place-cluster #10(w371) -> ("Config"=w386:T12)
              n192 = local read "Macro Name"() -> (w376:string)
              n193 = call-poly <vilib>:"Write Key.vi"("section"=w376, "error in (no error)"=w384, "value"=w383, "key"="data", "refnum"=w386) -> ("error out"=w381:errorcluster, "refnum out"=w382:T12)  [unwired: 4 in, 1 out]
              n194 = call <vilib>:"Close Config Data.vi"("error in (no error)"=w381, "refnum"=w382) -> ("error out"=w379:errorcluster, "file path"=w380:path)  [unwired: 8 in]
              n195 = call <vilib>:"Open Config Data.vi"("error in (no error)"=w379, "configuration file path"=w380) -> ("error out"=w377:errorcluster, "refnum"=w378:T12)  [unwired: 7 in, 1 out]
              n196 = in-place-cluster #10("Config"=w378) -> (w372:T13)
            }
          }
        }
      }
      frame "Data: Load Process" {
        n197 = local read "Macro Name"() -> (w407:string)
        n198 = Unbundle By Name(w392) -> ("Config"=w405:T12)
        n199 = call-poly <vilib>:"Read Key.vi"("section"=w407, "error in (no error)"=w406, "key"="data", "refnum"=w405) -> ("error out"=w402:errorcluster, "value"=w403:string, "found?"=w396:bool)  [unwired: 4 in, 1 out]
        n200 = case shown="False" w396 {
          tunnel: w403 -> [_ w420]
          tunnel: w402 -> [w412 w419]
          tunnel: [w412 w418] -> w401
          tunnel: [w409 w415] -> w399
          tunnel: [w408 w414] -> w398
          tunnel: [w410 w413] -> w394
          tunnel: w392 -> [w411 _]
          frame False {
            n201 = Unbundle By Name(w411) -> ("Steps"=w410:T7[])
            n202 = property on="Activation Type" class="RadioBtnsControl (strict)"() -> ("Value"=w409:enum32{"Hotkey", "Automatic"})  [unwired: 2 in, 2 out]
            n203 = property on="N" class="DigNum (strict)"() -> ("Value"=w408:i32)  [unwired: 2 in, 2 out]
          }
          frame True {
            n204 = Unflatten From String(type=T10 {"Steps"=[], "Activation Type"=enum."Hotkey", "N"=0} ("cluster"), binary string=w420, error in (no error)=w419) -> (value=w417:T10, error out=w418:errorcluster)  [unwired: 2 in, 1 out]
            n205 = Unbundle By Name(w417) -> ("Steps"=w413:T7[], "Activation Type"=w415:enum32{"Hotkey", "Automatic"}, "N"=w414:i32)
          }
        }
        n206 = call-poly <userlib>:"MGI Gray if.vi"("Boolean"=w396) -> ("Disabled"=w397:T6)
        n207 = property on="Restore" class="Bool"("DisabledEnum"=w397) -> ()  [unwired: 2 in, 2 out]
        n208 = property on="Activation Type" class="RadioBtnsControl (strict)"("Val(Sgnl)"=w399) -> ()  [unwired: 2 in, 2 out]
        n209 = property on="N" class="DigNum (strict)"("Val(Sgnl)"=w398) -> ()  [unwired: 2 in, 2 out]
        n210 = call "Enqueue Multiple States.vi"("queue in"=w395, "State(s) at Back"="UI: Display Process" ("State(s) at Back (\"\")")) -> ()  [unwired: 13 in, 1 out]
        n211 = Bundle By Name(cluster=w392, "Steps"=w394) -> (w393:T13)
      }
      frame "Data: Delete Process" {
        n212 = call "Perm Delete?"("error in (no error)"=w423) -> ("error out"=w424:errorcluster, "Delete"=w425:bool)  [unwired: 9 in]
        n213 = case shown="True" w425 {
          tunnel: w424 -> [w426 w433]
          tunnel: [w426 w428] -> w422
          tunnel: w421 -> [_ w432]
          frame False {
          }
          frame True {
            n214 = local read "Macro Name"() -> (w430:string)
            n215 = Unbundle By Name(w432) -> ("Config"=w431:T12)
            n216 = call <vilib>:"Remove Section.vi"("section"=w430, "error in (no error)"=w433, "refnum"=w431) -> ("error out"=w429:errorcluster)  [unwired: 6 in, 2 out]
            n217 = property on="Macro Name" class="CmbBox"(error in=w429, "Val(Sgnl)"="") -> (error out=w428:errorcluster)  [unwired: 1 in, 1 out]
          }
        }
      }
      frame "Data: Flush Queue" {
        n218 = Flush Queue(queue=w434) -> ()  [unwired: 1 in, 3 out]
      }
      frame "Data: Cleanup" {
        # "Cleanup any data and references, here.\n(this is called automatically, by the Macro: Exit)"
        n219 = Unbundle By Name(w444) -> ("Core.Current VI Reference"=w443:refnum<vi>, "Keyboard"=w437:refnum<k1>)
        n220 = Close Reference(reference=w443, error in (no error)=w441) -> (error out=w438:errorcluster)
        n221 = call-poly <vilib>:"Close Input Device.vi"("error in (no error)"=w438, "device ID"=w437) -> ("error out"=w439:errorcluster)  [unwired: 8 in]
        n222 = invoke class="VI" method="Default Vals.Reinit All"(error in=w439) -> (error out=w442:errorcluster)  [unwired: 2 in, 2 out]
        n223 = call "Enqueue Multiple States.vi"("queue in"=w440) -> ()  [unwired: 14 in, 1 out]
      }
      frame "---------- UI ----------" {
        # "Do not put any code in this frame.\n(It is a separator no-op. You can make a copy of this frame to create a new UI frame)"
        n224 = call "Enqueue Multiple States.vi"("queue in"=w445) -> ()  [unwired: 14 in, 1 out]
      }
      frame "UI: Initialize" {
        w455 = T6."Disabled and Grayed Out" ("Disabled")
        # "Initialize the User Interface, here.\n(this is called automatically, by the Macro: Init)"
        n225 = property on="Start/Stop" class="Bool (strict)"("DisabledEnum"=w455) -> ()  [unwired: 2 in, 2 out]
        n226 = property on="Restore" class="Bool"("DisabledEnum"=w455) -> ()  [unwired: 2 in, 2 out]
        n227 = property on="Save" class="Bool"("DisabledEnum"=w455) -> ()  [unwired: 2 in, 2 out]
        n228 = call "Hotkey FGV.vi"("error in (no error)"=w453) -> ("error out"=w452:errorcluster, "Hotkey String out"=→"Application Hotkey":string, "Hotkey out"=w448:T15)  [unwired: 8 in]
        n229 = Bundle By Name(cluster=w450, "Hotkey"=w448) -> (w449:T13)
        n230 = call "Enqueue Multiple States.vi"("queue in"=w454) -> ()  [unwired: 14 in, 1 out]
      }
      frame "UI: Cursor Set" {
        # "Argument"
        # "Set and Unset Cursor Busy.\n(Usage: \"UI: Cursor Set >> Busy|Idle\")"
        n231 = case shown="\"Idle\", Default" w457 {
          tunnel: w459 -> [w462 w464]
          tunnel: [w461 w463] -> w458
          frame "Idle", Default {
            n232 = call <vilib>:"Unset Busy.vi"("error in (no error)"=w462) -> ("error out"=w461:errorcluster)  [unwired: 10 in]
          }
          frame "Busy" {
            n233 = call <vilib>:"Set Busy.vi"("error in (no error)"=w464) -> ("error out"=w463:errorcluster)  [unwired: 9 in, 1 out]
          }
        }
        n234 = call "Enqueue Multiple States.vi"("queue in"=w456) -> ()  [unwired: 14 in, 1 out]
      }
      frame "UI: Front Panel State" {
        # "Argument"
        # "Set Front Panel Open or Closed\n(Usage: \"UI: Front Panel State >> Open|Close\")"
        n235 = Unbundle By Name(w468) -> ("Core.Current VI Reference"=w467:refnum<vi>)
        n236 = case shown="\"Hidden\", \"Hide\"" w466 {
          tunnel: w470 -> [w476 w491 w502 w515 w528]
          tunnel: [w478 w492 w504 w517 w530] -> w469
          tunnel: w467 -> [w477 w489 w503 w516 w529]
          frame "Open", "Standard", Default {
            w471 = T4."Standard" ("State")
            n237 = property class="VI"(reference=w477, error in=w476) -> (reference out=w474:refnum<vi>, error out=w475:errorcluster, "FP.State"=w473:T4)
            n238 = Not Equal?(x=w473, y=w471) -> (x != y?=w472:bool)
            n239 = case shown="False" w472 {
              tunnel: [w482 w484] -> w478
              tunnel: w475 -> [w481 w484]
              tunnel: w474 -> [w480 _]
              tunnel: w471 -> [w479 _]
              frame True {
                n240 = invoke class="VI" method="FP.Open"(reference=w480, error in=w481, "Activate"=TRUE, "State"=w479) -> (error out=w482:errorcluster)  [unwired: 1 in, 4 out]
              }
              frame False {
              }
            }
          }
          frame "Close", "Closed" {
            n241 = property class="VI"(reference=w489, error in=w491) -> (reference out=w488:refnum<vi>, error out=w490:errorcluster, "FP.State"=w486:T4)
            n242 = Not Equal?(x=w486, y=T4."Closed" ("Front Panel Window:State")) -> (x != y?=w485:bool)
            n243 = case shown="True" w485 {
              tunnel: [w493 w496] -> w492
              tunnel: w490 -> [w493 w495]
              tunnel: w488 -> [_ w494]
              frame False {
              }
              frame True {
                n244 = invoke class="VI" method="FP.Close"(reference=w494, error in=w495) -> (error out=w496:errorcluster)  [unwired: 1 in, 2 out]
              }
            }
          }
          frame "Hidden", "Hide" {
            w497 = T4."Hidden" ("State")
            n245 = property class="VI"(reference=w503, error in=w502) -> (reference out=w500:refnum<vi>, error out=w501:errorcluster, "FP.State"=w499:T4)
            n246 = Not Equal?(x=w499, y=w497) -> (x != y?=w498:bool)
            n247 = case shown="True" w498 {
              tunnel: [w508 w509] -> w504
              tunnel: w501 -> [w507 w509]
              tunnel: w500 -> [w506 _]
              tunnel: w497 -> [w505 _]
              frame True {
                n248 = invoke class="VI" method="FP.Open"(reference=w506, error in=w507, "State"=w505) -> (error out=w508:errorcluster)  [unwired: 2 in, 4 out]
              }
              frame False {
              }
            }
          }
          frame "Minimize", "Minimized" {
            w510 = T4."Minimized" ("State")
            n249 = property class="VI"(reference=w516, error in=w515) -> (reference out=w513:refnum<vi>, error out=w514:errorcluster, "FP.State"=w512:T4)
            n250 = Not Equal?(x=w512, y=w510) -> (x != y?=w511:bool)
            n251 = case shown="True" w511 {
              tunnel: [w521 w522] -> w517
              tunnel: w514 -> [w520 w522]
              tunnel: w513 -> [w519 _]
              tunnel: w510 -> [w518 _]
              frame True {
                n252 = invoke class="VI" method="FP.Open"(reference=w519, error in=w520, "State"=w518) -> (error out=w521:errorcluster)  [unwired: 2 in, 4 out]
              }
              frame False {
              }
            }
          }
          frame "Maximize", "Maximized" {
            w523 = T4."Maximized" ("State")
            n253 = property class="VI"(reference=w529, error in=w528) -> (reference out=w526:refnum<vi>, error out=w527:errorcluster, "FP.State"=w525:T4)
            n254 = Not Equal?(x=w525, y=w523) -> (x != y?=w524:bool)
            n255 = case shown="True" w524 {
              tunnel: [w534 w535] -> w530
              tunnel: w527 -> [w533 w535]
              tunnel: w526 -> [w532 _]
              tunnel: w523 -> [w531 _]
              frame True {
                n256 = invoke class="VI" method="FP.Open"(reference=w532, error in=w533, "State"=w531) -> (error out=w534:errorcluster)  [unwired: 2 in, 4 out]
              }
              frame False {
              }
            }
          }
        }
        n257 = call "Enqueue Multiple States.vi"("queue in"=w465) -> ()  [unwired: 14 in, 1 out]
      }
      frame "UI: Populate Processes" {
        n258 = Unbundle By Name(w540) -> ("Config"=w537:T12)
        n259 = call <vilib>:"Get Section Names.vi"("error in (no error)"=w539, "refnum"=w537) -> ("error out"=w538:errorcluster, "section names"=w536:string[])  [unwired: 7 in, 1 out]
        n260 = property on="Macro Name" class="CmbBox"("Strings[]"=w536) -> ()  [unwired: 2 in, 2 out]
      }
      frame "UI: Display Process" {
        n261 = Unbundle By Name(w554) -> ("Steps"=w550:T7[])
        n262 = local read "Macro Name"() -> (w548:string)
        n263 = Empty Array?(array=w550) -> (empty?=w549:bool)
        n264 = Empty String/Path?(string/path=w548) -> (empty?=w547:bool)
        n265 = Not(x=w547) -> (.not. x?=w546:bool)
        n266 = Not(x=w549) -> (.not. x?=w543:bool)
        n267 = And(x=w546, y=w543) -> (x .and. y?=w545:bool)
        n268 = call-poly <userlib>:"MGI Gray if.vi"("Boolean"=w545) -> ("Disabled"=w544:T6)
        n269 = call-poly <userlib>:"MGI Gray if.vi"("Boolean"=w543) -> ("Disabled"=w542:T6)
        n270 = call "Display Data to Table.vi"("error in (no error)"=w552, "Test Data In"=w550) -> ("error out"=w551:errorcluster, "Array"=→"Table":string[][])  [unwired: 8 in]
        n271 = property on="Save" class="Bool"("DisabledEnum"=w544) -> ()  [unwired: 2 in, 2 out]
        n272 = property on="Start/Stop" class="Bool (strict)"("DisabledEnum"=w542) -> ()  [unwired: 2 in, 2 out]
        n273 = call "Enqueue Multiple States.vi"("queue in"=w541) -> ()  [unwired: 14 in, 1 out]
      }
      frame "UI: Refs" {
        n274 = Unbundle By Name(w558) -> ("Refs"=w556:refnum<vi>[])
        n275 = case shown="\"Disable\", Default" w559 {
          tunnel: [FALSE TRUE] -> _
          tunnel: [T6."Disabled and Grayed Out" ("Enum Out") T6."Enabled" ("Disabled")] -> w555
          frame "Disable", Default {
          }
          frame "Enable" {
          }
        }
        n276 = for {
          tunnel: w556 -> [w561] mode=indexing
          tunnel: w555 -> [w560]
          n277 = property class="Ctl"(reference=w561, "DisabledEnum"=w560) -> ()  [unwired: 1 in, 2 out]
        }
      }
      frame "UI: Wait" {
        n278 = call "Timer FGV.vi"("Mode"=FGV_Actions."Read", "error in (no error)"=w570) -> ("error out"=w573:errorcluster, "Expired?"=w571:bool)  [unwired: 7 in, 1 out]
        n279 = Select(t="Macro: Process >> Step", s=w571, f="UI: Wait") -> (s? t:f=w567:string)
        n280 = call "Enqueue Multiple States.vi"("queue in"=w566, "State(s) at Back"=w567) -> ()  [unwired: 13 in, 1 out]
      }
      frame "UI: Listen" {
        n281 = Unbundle By Name(w579) -> ("Hotkey"=w575:T15, "Keyboard"=w588:refnum<k1>)
        n282 = call "Stall Data Flow.vim"("value in"=w588, "milliseconds to wait"=u32 1) -> ("value out"=w583:refnum<k1>)  [unwired: 1 out]
        n283 = call-poly <vilib>:"Acquire Input Data.vi"("device ID"=w583, "error in (no error)"=w581) -> ("keys pressed"=w587:T15, "error out"=w580:errorcluster)  [unwired: 15 in, 1 out]
        n284 = Sort 1D Array(array=w587) -> (sorted array=w586:T15)
        n285 = Equal?(x=w575, y=w586) -> (x = y?=w585:bool)
        n286 = Select(t="Macro: Process >> Start", s=w585, f="UI: Listen" ("string")) -> (s? t:f=w578:string)
        n287 = call "Enqueue Multiple States.vi"("queue in"=w576, "State(s) at Back"=w578) -> ()  [unwired: 13 in, 1 out]
      }
      frame "UI: Settings" {
        n288 = call "Settings.vi"("error in (no error)"=w590) -> ("error out"=w589:errorcluster)  [unwired: 10 in]
      }
      frame "---------- Macro ----------" {
        # "Do not put any code in this frame.\n(It is a separator no-op. You can make a copy of this frame to create a new Macro frame)"
        n289 = call "Enqueue Multiple States.vi"("queue in"=w592) -> ()  [unwired: 14 in, 1 out]
      }
      frame "Macro: Initialize" {
        w596 = "Data: Initialize\nInitialize Core Data\nUI: Refs >> Enable\nUI: Initialize\nData: Open Config\nUI: Populate Processes\nUI: Front Panel State >> Open"  # Data: Initialize Initialize Core Data UI: Refs >> Enable UI: Initialize Data: Open Config UI: Populate Processes UI: Front Panel State >> Open
        # "Initialization Macro\n(This is called once, when the VI starts)"
        n290 = call "Enqueue Multiple States.vi"("State(s) at Front"=w596, "queue in"=w595) -> ()  [unwired: 13 in, 1 out]
      }
      frame "Macro: Process" {
        n291 = case shown="\"Start\", Default" w603 {
          tunnel: w599 -> [w608 w612 w617 w632 w636]
          tunnel: [w607 w611 w615 w630 w636] -> w602
          tunnel: ["Process: Perform Step" "Process: Perform Step" w613 w628 w635] -> w601
          frame "Start", Default {
            w605 = 0 ("Step")
            n292 = Bundle By Name(cluster=w608, "Step"=w605, "n"=w605) -> (w607:T13)
          }
          frame "Repeat" {
            n293 = Bundle By Name(cluster=w612, "Step"=0) -> (w611:T13)
          }
          frame "Step" {
            n294 = Unbundle By Name(w617) -> ("Step"=w622:i32, "Steps"=w620:T7[])
            n295 = Array Size(array=w620) -> (size(s)=w621:i32)
            n296 = Increment(x=w622) -> (x+1=w616:i32)
            n297 = Greater Or Equal?(x=w616, y=w621) -> (x >= y?=w619:bool)
            n298 = Select(t="Macro: Process >> Complete", s=w619, f="Process: Perform Step") -> (s? t:f=w613:string)
            n299 = Bundle By Name(cluster=w617, "Step"=w616) -> (w615:T13)
          }
          frame "Complete" {
            n300 = Unbundle By Name(w632) -> ("n"=w634:i32)
            n301 = Increment(x=w634) -> (x+1=w631:i32)
            n302 = local read "N"() -> (w627:i32)
            n303 = Greater?(x=w631, y=w627) -> (0:w625:bool)
            n304 = Not Equal?(x=w627, y=-1) -> (x != y?=w624:bool)
            n305 = And(x=w625, y=w624) -> (x .and. y?=w623:bool)
            n306 = Select(t="Macro: Process >> End", s=w623, f="Macro: Process >> Repeat") -> (s? t:f=w628:string)
            n307 = Bundle By Name(cluster=w632, "n"=w631) -> (w630:T13)
          }
          frame "End" {
            n308 = local read "Activation Type"() -> (w639:enum32{"Hotkey", "Automatic"})
            n309 = Equal?(x=w639, y=enum32{"Hotkey", "Automatic"}."Hotkey") -> (x = y?=w637:bool)
            n310 = case shown="False" w637 {
              tunnel: [_ "UI: Listen"] -> w635
              frame False {
                n311 = property on="Start/Stop" class="Bool (strict)"("Val(Sgnl)"=FALSE ("Value (Signaling)")) -> ()  [unwired: 2 in, 2 out]
              }
              frame True {
              }
            }
          }
        }
        n312 = call "Enqueue Multiple States.vi"("queue in"=w600, "State(s) at Back"=w601) -> ()  [unwired: 13 in, 1 out]
      }
      frame "Macro: Exit" {
        # "Exit Macro\n(This is called once, when the VI exits)"
        n313 = Unbundle By Name(w649) -> ("Core.Close Panel on Exit?"=w648:bool)
        n314 = property on="Table" class="Tbl (strict)"("Index Values"=T9 {"Row"=0, "Column"=0}) -> ()  [unwired: 2 in, 2 out]
        n315 = Select(t="UI: Front Panel State >> Close", s=w648, f="") -> (s? t:f=w643:string)
        n316 = call "Enqueue Multiple States.vi"("State(s) at Front"=w643, "queue in"=w644, "State(s) at Back"="Data: Cleanup\nExit") -> ()  [unwired: 12 in, 1 out]
      }
      frame "---------- Process ----------" {
        n317 = call "Enqueue Multiple States.vi"("queue in"=w651) -> ()  [unwired: 14 in, 1 out]
      }
      frame "Process: Perform Step" {
        n318 = Unbundle By Name(w671) -> ("Steps"=w670:T7[], "Step"=w669:i32)
        n319 = Index Array(array=w670, index=w669) -> (element=w668:T7)
        n320 = Unbundle By Name(w668) -> ("Repeat"=w658:i32, "Type"=w667:T8, "Coords"=w666:cluster{"x":i32, "y":i32}, "Delay"=w665:i32, "Key"=w664:u8, "RClick?"=w660:bool)
        n321 = Increment(x=w658) -> (x+1=w657:i32)
        n322 = Equal To 0?(x=w657) -> (x = 0?=w659:bool)
        n323 = Select(t=2147483647, s=w659, f=w657) -> (s? t:f=w656:i32)
        n324 = for {
          N: w656 -> [_]
          tunnel: w667 -> [w679]
          tunnel: w666 -> [w678]
          tunnel: w665 -> [w677]
          tunnel: w664 -> [w676]
          tunnel: [w673] -> w661
          tunnel: w660 -> [w672]
          shift-right: [w674] -> w662
          shift-left: w663 -> [w675]
          n325 = case shown="\"Mouse Click\"" w679 {
            tunnel: w678 -> [w686 _ _ _ _ _ _ _]
            tunnel: w677 -> [w683 w692 w702 w706 w711 w717 w722 w728]
            tunnel: w676 -> [_ _ w697 _ _ w716 w721 _]
            tunnel: w675 -> [w687 w695 w704 w709 w714 w719 w724 w731]
            tunnel: [w684 w694 w703 w708 w713 w718 w723 w730] -> w674
            tunnel: ["Macro: Process >> Step" "Macro: Process >> Step" "Macro: Process >> Step" "Macro: Process >> Step" "Macro: Process >> Step" "Macro: Process >> Step" "Macro: Process >> Step" "UI: Wait"] -> w673
            tunnel: w672 -> [_ w693 _ w707 w712 _ _ _]
            frame "Mouse Move", Default {
              n326 = Unbundle By Name(w686) -> ("x"=w682:i32, "y"=w681:i32)
              n327 = call "Mouse Move.vi"("error in (no error)"=w687, "y"=w681, "x"=w682) -> ("error out"=w685:errorcluster)  [unwired: 8 in]
              n328 = call "Stall Data Flow.vim"("value in"=w685, "milliseconds to wait"=w683) -> ("value out"=w684:errorcluster)  [unwired: 1 out]
            }
            frame "Mouse Click" {
              n329 = Quotient & Remainder(x=w692, y=2) -> (x-y*floor(x/y)=w690:i32, floor(x/y)=w688:i32)
              n330 = Add(x=w690, y=w688) -> (x+y=w689:i32)
              n331 = call "Mouse Click.vi"("error in (no error)"=w695, "ms wait after up (10)"=w689, "ms wait after down (10)"=w688, "Right Click? (F)"=w693) -> ("error out"=w694:errorcluster)  [unwired: 7 in]
            }
            frame "Key Press" {
              n332 = Quotient & Remainder(x=w702, y=2) -> (x-y*floor(x/y)=w700:i32, floor(x/y)=w698:i32)
              n333 = Add(x=w700, y=w698) -> (x+y=w699:i32)
              n334 = call "Key Press.vi"("error in (no error)"=w704, "ms wait after up (20)"=w699, "ms wait after down (80)"=w698, "Virtual Key"=w697) -> ("error out"=w703:errorcluster)  [unwired: 7 in]
            }
            frame "Mouse Down" {
              n335 = call "Mouse Down.vi"("error in (no error)"=w709, "Delay in ms (10)"=w706, "Right Click? (F)"=w707) -> ("error out"=w708:errorcluster)  [unwired: 8 in]
            }
            frame "Mouse Up" {
              n336 = call "Mouse Up.vi"("error in (no error)"=w714, "Delay in ms (10)"=w711, "Right Click? (F)"=w712) -> ("error out"=w713:errorcluster)  [unwired: 8 in]
            }
            frame "Key Down" {
              n337 = call "Key Down.vi"("error in (no error)"=w719, "delay in ms (80)"=w717, "Virtual Key"=w716) -> ("error out"=w718:errorcluster)  [unwired: 8 in]
            }
            frame "Key Up" {
              n338 = call "Key Up.vi"("error in (no error)"=w724, "delay in ms (20)"=w722, "Virtual Key"=w721) -> ("error out"=w723:errorcluster)  [unwired: 8 in]
            }
            frame "Wait" {
              n339 = Divide(x=w728, y=1000) -> (x/y=w726:dbl)
              n340 = call "Timer FGV.vi"("Mode"=FGV_Actions."Write", "error in (no error)"=w731, "Timer Value (s)"=w726) -> ("error out"=w730:errorcluster)  [unwired: 6 in, 2 out]
            }
          }
        }
        n341 = call "Enqueue Multiple States.vi"("queue in"=w655, "State(s) at Back"=w661) -> ()  [unwired: 13 in, 1 out]
      }
    }
  }
  n342 = Merge Errors(w9, w8) -> (w10:errorcluster)
  n343 = Release Queue(queue=w11, error in (no error)=w10) -> (error out=→"error out":errorcluster)  [unwired: 1 in, 2 out]
